vi "b2g1_sqlite_log_time.vi"(8 "error in (no error)":errorcluster, 9 "nd_vars out in":T1, 10 "Output - Cluster b2g1":T2 {"TS-6 [°C]" format="%#.2g"; "TS-5 [°C]" format="%#.2g"; "pHS-1 [pH]" format="%.2g"; "TS-4 [°C]" format="%#.2g"; "FS-2 [l]" format="%.2g"; "FS-1 [l]" format="%.2g"; "DS-1 [bar]" format="%#.2g"; "DFS-1 [l/min]" format="%#.2g"; "FS-3 [l]" format="%.2g"; "DFS-1 [dl]" format="%.0g"}, 11 "Actual Start [f]":i64) -> (0 "error out":errorcluster, 3 "nd_vars out out":T1)   [LabVIEW 2011]
uses:
  B2G1_nd_vars.ctl
  Output - Cluster b2g1.ctl
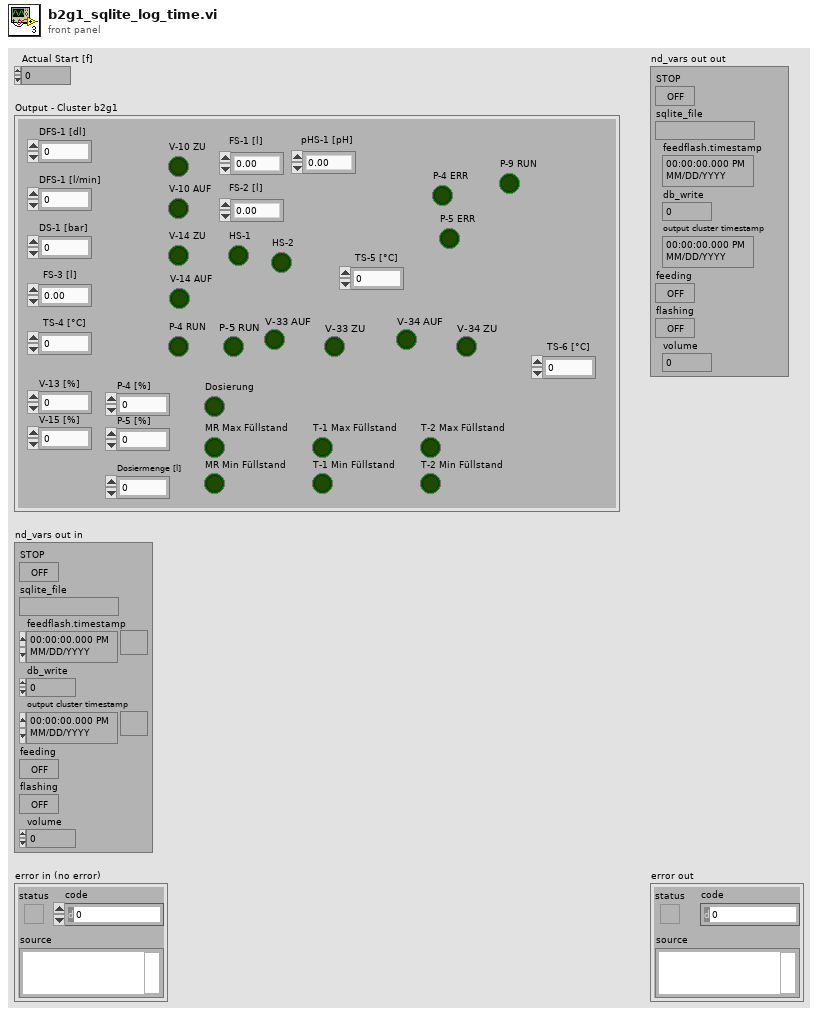
[diagram p1: front panel]
types:
  T1 = typedef "B2G1_nd_vars.ctl" = cluster{"STOP":bool, "sqlite_file":string, "feedflash.timestamp":timestamp, "db_write":i64, "output cluster timestamp":timestamp, "feeding":bool, "flashing":bool, "volume":u64}
  T2 = typedef "Output - Cluster b2g1.ctl" = cluster{"DFS-1 [dl]":u64, "FS-3 [l]":dbl, "DFS-1 [l/min]":dbl, "DS-1 [bar]":dbl, "V-10 ZU":bool, "V-14 ZU":bool, "FS-1 [l]":dbl, "FS-2 [l]":dbl, "TS-4 [°C]":dbl, "HS-1":bool, "V-13 [%]":u8, "V-15 [%]":u8, "P-4 [%]":u8, "P-5 [%]":u8, "Dosierung":bool, "MR Max Füllstand":bool, "MR Min Füllstand":bool, "Dosiermenge [l]":sgl, "V-14 AUF":bool, "V-10 AUF":bool, "T-1 Max Füllstand":bool, "T-1 Min Füllstand":bool, "T-2 Max Füllstand":bool, "T-2 Min Füllstand":bool, "pHS-1 [pH]":dbl, "P-4 RUN":bool, "P-5 RUN ":bool, "V-33 AUF":bool, "V-33 ZU":bool, "V-34 AUF":bool, "V-34 ZU":bool, "P-4 ERR":bool, "P-5 ERR":bool, "TS-5 [°C]":dbl, "TS-6 [°C]":dbl, "P-9 RUN":bool, "HS-2":bool}
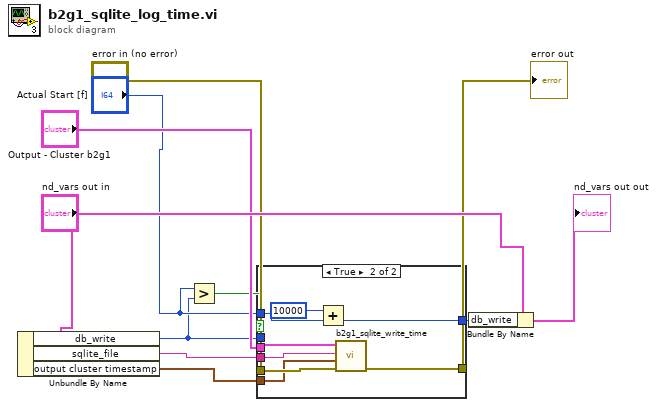
[diagram p0: block diagram]
diagram:
  n1 = Unbundle By Name("nd_vars out in") -> ("db_write"=w5:i64, "sqlite_file"=w3:string, "output cluster timestamp"=w4:timestamp)
  n2 = Greater?(x="Actual Start [f]", y=w5) -> (0:w2:bool)
  n3 = case shown="True" w2 {
    tunnel: "Actual Start [f]" -> [_ w21]
    tunnel: w5 -> [w13 _]
    tunnel: [w13 w20] -> w1
    tunnel: "error in (no error)" -> [w12 w18]
    tunnel: [w12 w17] -> w7
    tunnel: w3 -> [_ w16]
    tunnel: w4 -> [_ w15]
    tunnel: "Output - Cluster b2g1" -> [_ w14]
    frame False {
    }
    frame True {
      n4 = Add(x=i64 10000, y=w21) -> (x+y=w20:i64)
      n5 = call "b2g1_sqlite_write_time.vi"("error in (no error)"=w18, "output cluster timestamp"=w15, "Database File"=w16, "Output - Cluster b2g1"=w14) -> ("error out"=w17:errorcluster)  [unwired: 7 in]
    }
  }
  "error out" <- w7
  n6 = Bundle By Name(cluster="nd_vars out in", "db_write"=w1) -> (→"nd_vars out out":T1)
